vi "shutdown.vi"(8 "error in":errorcluster, 11 "http responder in":refnum<class "http responder.lvclass">) -> (0 "error out":errorcluster)   [LabVIEW 2016, in "http responder.lvclass"]
uses:
  http responder.lvclass
  http responder.lvclass/http responder.ctl
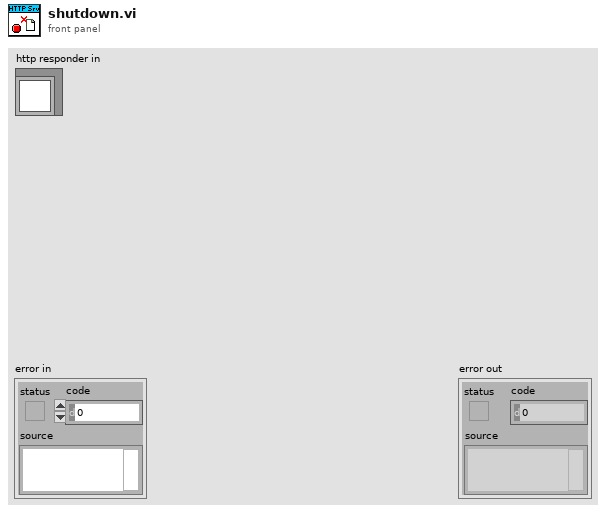
[diagram p1: front panel]
types:
  T1 = typedef "http responder.lvclass/http plugins.ctl" = cluster{"name":string[], "callbacks":T2[]}
  T2 = typedef "http responder.lvclass/http upgrade callback.ctl" = cluster{"callback":refnum<vi>, "parameters":variant, "unregister callback":refnum<vi>}
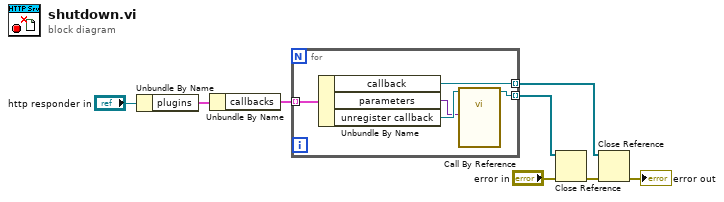
[diagram p0: block diagram]
diagram:
  n1 = Unbundle By Name("http responder in") -> ("plugins"=w5:T1)
  n2 = Unbundle By Name(w5) -> ("callbacks"=w7:T2[])
  n3 = for {
    tunnel: w7 -> [w13] mode=indexing
    tunnel: [w12] -> w6 mode=indexing
    tunnel: [w9] -> w1 mode=indexing
    n4 = Unbundle By Name(w13) -> ("callback"=w12:refnum<vi>, "parameters"=w10:variant, "unregister callback"=w11:refnum<vi>)
    n5 = call-by-ref "?"(reference=w11, "parameters"=w10) -> (reference out=w9:refnum<vi>)  [unwired: 12 in, 1 out]
  }
  n6 = Close Reference(reference=w1, error in (no error)="error in") -> (error out=w2:errorcluster)
  n7 = Close Reference(reference=w6, error in (no error)=w2) -> (error out=→"error out":errorcluster)
